vi "distribute_setpoints_DC.vi"(8 "setpoints":dbl[](array[numeric])) -> (2 "reference_DC":T1)   [LabVIEW 2021]
uses:
  controls/SC_references.ctl
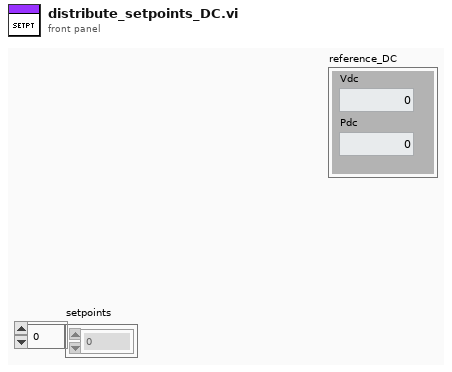
[diagram p1: front panel]
types:
  T1 = typedef "SC_references.ctl" = cluster{"Vdc":dbl, "Pdc":dbl}
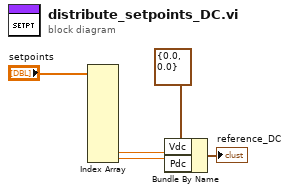
[diagram p0: block diagram]
diagram:
  n1 = Index Array(array="setpoints") -> (element #9=w2:dbl, element #10=w1:dbl)  [unwired: 10 in, 8 out]
  n2 = Bundle By Name(cluster=T1 {"Vdc"=0.0, "Pdc"=0.0} ("SC references"), "Vdc"=w2, "Pdc"=w1) -> (→"reference_DC":T1)
